vi "BasicValueVI.vi"() -> ()   [LabVIEW 2018]
panel:
  in  "Value":u64
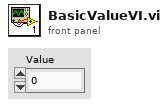
[diagram p1: front panel]
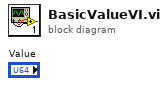
[diagram p0: block diagram]
diagram:
